vi "emi_New Loop.vi"   [LabVIEW 2010]
doc: "Create New Lopp. Eiterh a single on, using a single ID, or several linked once using an array.\n\nLinked loops needs all to be started, and an error ion one will restart them all"
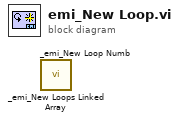
[diagram p0: block diagram]
diagram:
  n1 = call "_emi_New Loops Linked Array.vi"() -> ()  [unwired: 14 in, 2 out]
  n2 = call "_emi_New Loop Numb.vi"() -> ()  [unwired: 14 in, 2 out]
